vi "PROIECTU2.vi"() -> ()   [LabVIEW 2015]
uses:
  <vilib>/picture/picture.llb/Draw True-Color Pixmap.vi
panel:
  in  "Destinatia1":path
  out "new":u32[][](array[numeric]) format="%x"
  out "new picture":picture
  in  "Imaginea1":path
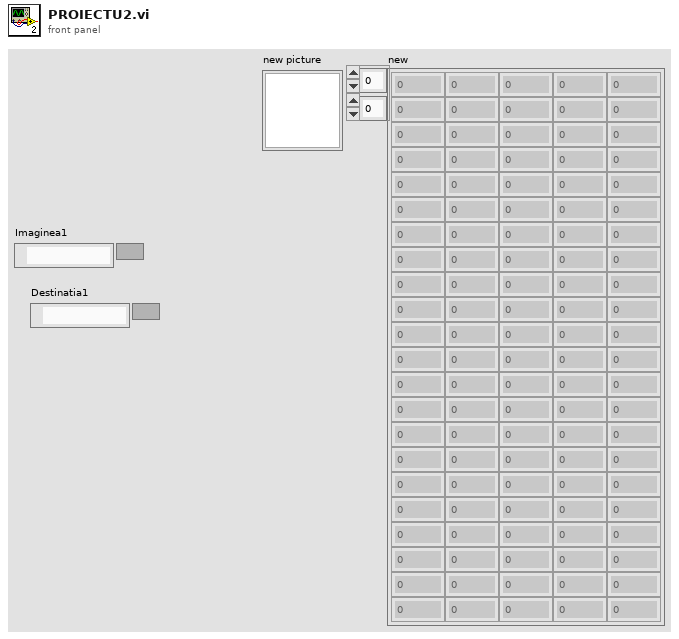
[diagram p1: front panel]
types:
  T1 = typedef "imagedata.ctl" = cluster{"image type":i32, "image depth":i32, "image":u8[], "mask":u8[], "colors":u32[], "Rectangle":cluster{"left":i16, "top":i16, "right":i16, "bottom":i16}}
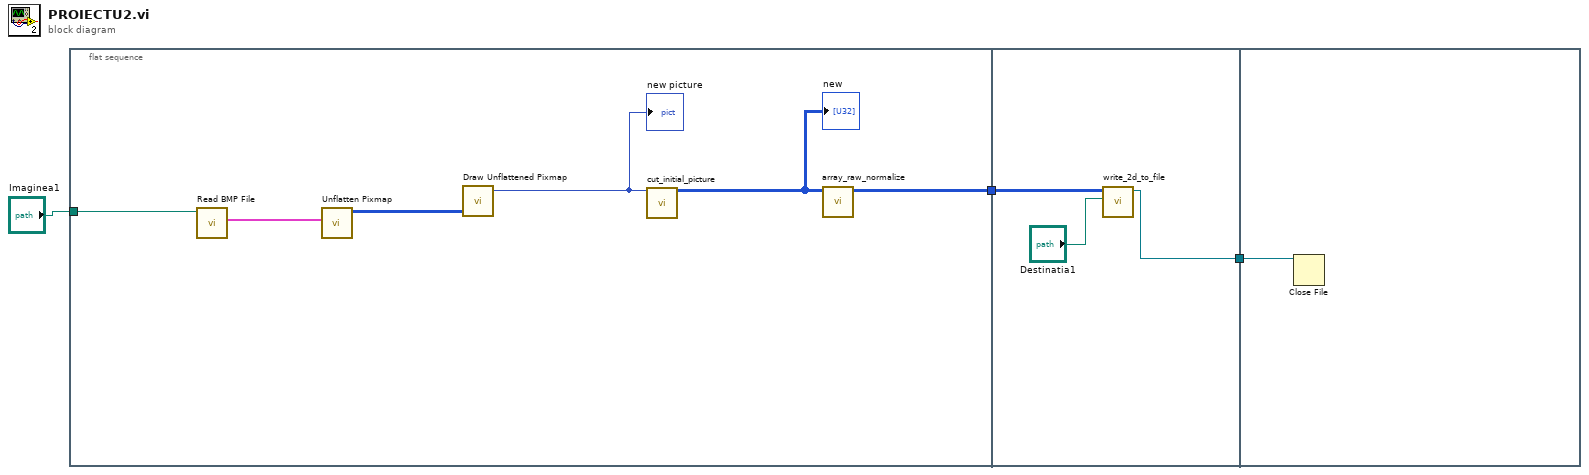
[diagram p0: block diagram]
diagram:
  n1 = flat-sequence {
    tunnel: [w5] -> w3
    tunnel: "Imaginea1" -> [w4]
    tunnel: w3 -> [w12]
    tunnel: [w10] -> w2
    tunnel: w2 -> [w13]
    frame #0 {
      n2 = call <vilib>:"Read BMP File.vi"("path to BMP file"=w4) -> ("image data"=w6:T1)  [unwired: 8 in, 2 out]
      n3 = call <vilib>:"Unflatten Pixmap.vi"("image data"=w6) -> ("24-bit pixmap"=w7:u32[][])  [unwired: 4 in, 6 out]
      n4 = call-poly <vilib>:"Draw Unflattened Pixmap.vi"("data (RGB format)"=w7) -> ("new picture"=w8:picture)  [unwired: 8 in]
      "new picture" <- w8
      n5 = call "cut_initial_picture.vi"("picture"=w8) -> ("new"=w9:u32[][])  [unwired: 14 in]
      "new" <- w9
      n6 = call "array_raw_normalize.vi"("array"=w9) -> ("Array"=w5:u8[][])  [unwired: 10 in]
    }
    frame #1 {
      n7 = call "write_2d_to_file.vi"("Path 2"="Destinatia1", "Array"=w12) -> ("refnum out"=w10:refnum<file>)  [unwired: 9 in]
    }
    frame #2 {
      n8 = Close File(refnum=w13) -> ()  [unwired: 1 in, 2 out]
    }
  }
